vi "while_v0_v5.vi"() -> ()   [LabVIEW 2009]
panel:
  out "Waveform Chart":dbl(graph)=0.6819636200681356
  in  "stop":bool
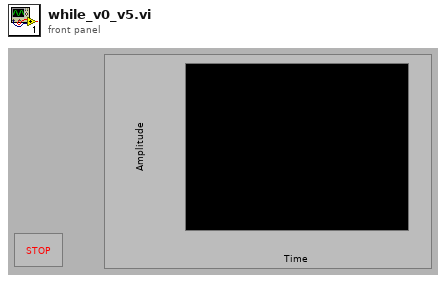
[diagram p1: front panel]
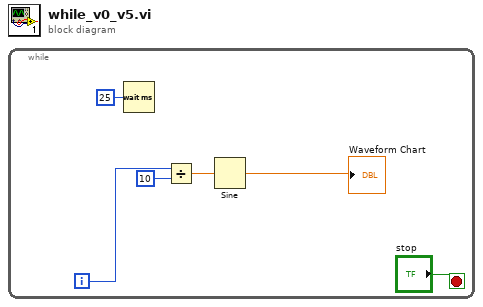
[diagram p0: block diagram]
diagram:
  n1 = while {
    i -> [w4]
    stop <- "stop" stop-if-true
    n2 = Wait (ms)(milliseconds to wait=u32 25) -> ()  [unwired: 1 out]
    n3 = Divide(x=w4, y=10) -> (x/y=w5:dbl)
    n4 = Sine(x=w5) -> (sin(x)=→"Waveform Chart":dbl)
  }
